vi "Scripting_GetControlFromTypeDef.vi"(0 "TypeDefControl":path=path "C:/classes/ObjectAttributes.ctl", 1 "String":string="Base class.Base class.Attribute1", 5 "error in":errorcluster, 6 "AppRef":refnum<vi>) -> (14 "vi reference":refnum<vi>, 15 "Panel":refnum<vi>, 16 "ControlRef":refnum<vi>, 19 "error out":errorcluster)   [LabVIEW 2020]
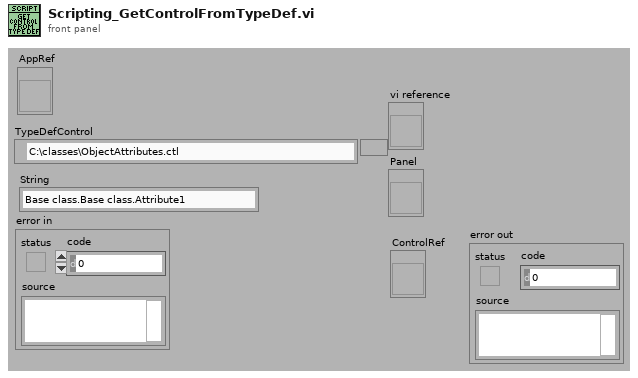
[diagram p1: front panel]
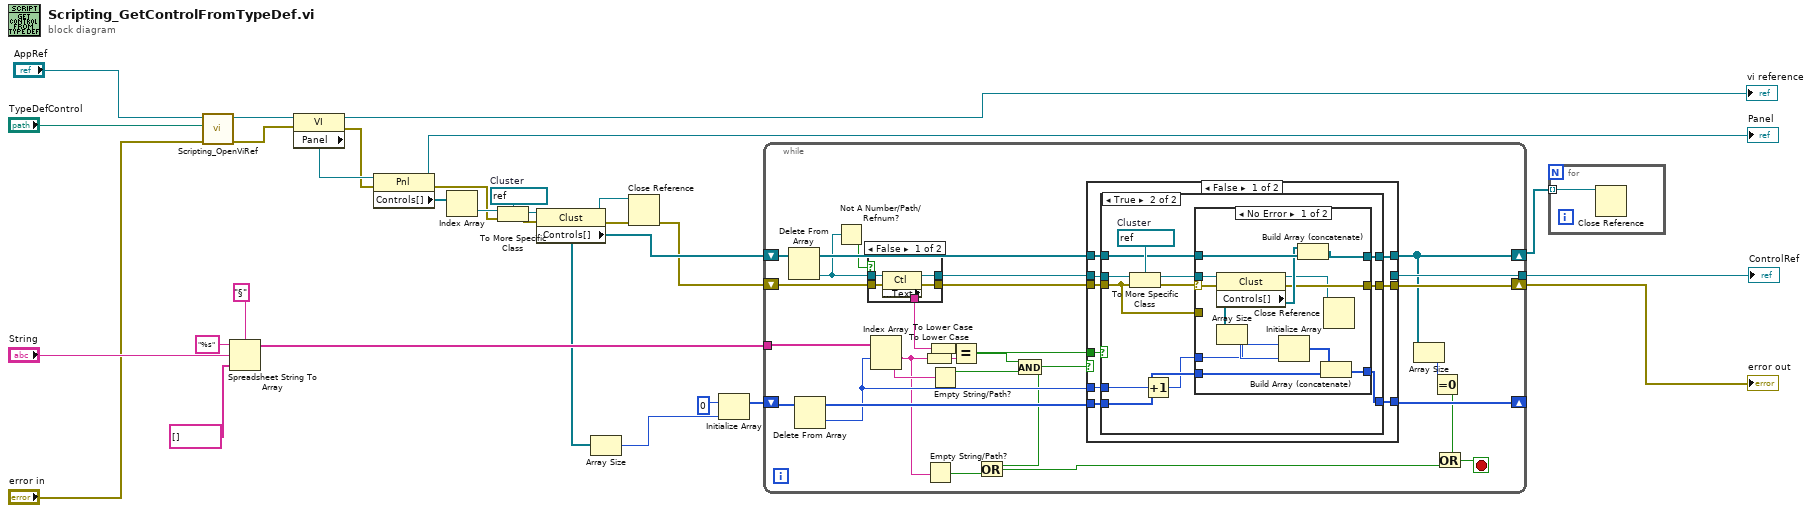
[diagram p0: block diagram]
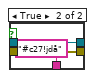
[diagram p2: hidden frame]
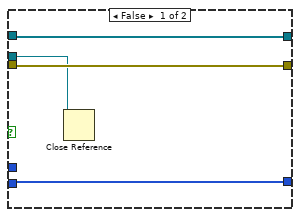
[diagram p3: hidden frame]
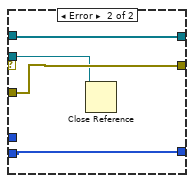
[diagram p4: hidden frame]
diagram:
  w27 = refnum<vi> refnum  # Cluster
  n1 = call <resource>:"Scripting_OpenViRef.vi"("error in"="error in", "ViPath/ViName/Viref"="TypeDefControl", "AppRef"="AppRef") -> ("error out"=w7:errorcluster, "vi reference"=w8:refnum<vi>)  [unwired: 6 in, 1 out]
  n2 = Spreadsheet String To Array(delimiter (Tab)="§", format string="%s", spreadsheet string="String", array type (2D Dbl)=string[] []) -> (array=w21:string[])
  n3 = property class="VI"(reference=w8, error in=w7) -> (reference out=→"vi reference":refnum<vi>, error out=w11:errorcluster, "Panel"=w30:refnum<vi>)
  n4 = property class="Pnl"(reference=w30, error in=w11) -> (reference out=→"Panel":refnum<vi>, error out=w10:errorcluster, "Controls[]"=w29:refnum<vi>[])
  n5 = Index Array(array=w29) -> (element=w28:refnum<vi>)  [unwired: 1 in]
  n6 = To More Specific Class(target class=w27, reference=w28, error in=w10) -> (specific class reference=w26:refnum<vi>, error out=w9:errorcluster)
  n7 = property class="Clust"(reference=w26, error in=w9) -> (reference out=w13:refnum<vi>, error out=w14:errorcluster, "Controls[]"=w17:refnum<vi>[])
  n8 = Array Size(array=w17) -> (size(s)=w16:i32)
  n9 = Close Reference(reference=w13, error in (no error)=w14) -> (error out=w2:errorcluster)
  n10 = Initialize Array(0, w16) -> (w19:i32[])
  n11 = while {
    shift-right: [w38] -> w15
    shift-left: w17 -> [w58]
    tunnel: w21 -> [w57]
    shift-right: [w48] -> _
    shift-left: w19 -> [w51]
    tunnel: [w52] -> w20
    shift-right: [w41] -> w3
    shift-left: w2 -> [w43]
    stop <- w39 stop-if-true
    n12 = Delete From Array(array=w58) -> (deleted portion=w35:refnum<vi>, array with subset deleted=w54:refnum<vi>[])  [unwired: 2 in]
    n13 = Delete From Array(array=w51) -> (deleted portion=w49:i32, array with subset deleted=w50:i32[])  [unwired: 2 in]
    n14 = Not A Number/Path/Refnum?(number/path/refnum=w35) -> (NaN/Path/Refnum?=w34:bool)
    n15 = case shown="False" w34 {
      tunnel: [w63 "#c27!jdå" ("Label.Text")] -> w33
      tunnel: [w62 w66] -> w53
      tunnel: w43 -> [w61 w65]
      tunnel: [w60 w65] -> w42
      tunnel: w35 -> [w59 w66]
      frame False {
        n16 = property class="Ctl"(reference=w59, error in=w61) -> (reference out=w62:refnum<vi>, error out=w60:errorcluster, "Label.Text"=w63:string)
      }
      frame True {
      }
    }
    n17 = Index Array(array=w57, index #1=w49) -> (element #1=w46:string, element #2=w56:string)  [unwired: 1 in]
    n18 = To Lower Case(string=w46) -> (all lower case string=w31:string)
    n19 = Empty String/Path?(string/path=w46) -> (empty?=w45:bool)
    n20 = To Lower Case(string=w33) -> (all lower case string=w32:string)
    n21 = Empty String/Path?(string/path=w56) -> (empty?=w55:bool)
    n22 = Equal?(x=w32, y=w31) -> (x = y?=w44:bool)
    n23 = And(x=w44, y=w55) -> (x .and. y?=w47:bool)
    n24 = Or(x=w47, y=w45) -> (x .or. y?=w40:bool)
    n25 = case shown="False" w47 {
      tunnel: w54 -> [w74 w111]
      tunnel: [w73 w111] -> w38
      tunnel: w53 -> [w75 w110]
      tunnel: [_ w110] -> w52
      tunnel: w50 -> [w72 w109]
      tunnel: w49 -> [w71 _]
      tunnel: [w70 w109] -> w48
      tunnel: w44 -> [w69 _]
      tunnel: w42 -> [w68 w108]
      tunnel: [w67 w108] -> w41
      frame False {
        n26 = case shown="True" w69 {
          tunnel: w75 -> [w76 w90]
          tunnel: w74 -> [w79 w87]
          tunnel: [w79 w86] -> w73
          tunnel: w72 -> [w78 w85]
          tunnel: w71 -> [_ w84]
          tunnel: [w78 w82] -> w70
          tunnel: w68 -> [w77 w80]
          tunnel: [w77 w81] -> w67
          frame False {
            n27 = Close Reference(reference=w76) -> ()  [unwired: 1 in, 1 out]
          }
          frame True {
            w91 = refnum<vi> refnum  # Cluster
            n28 = To More Specific Class(target class=w91, reference=w90, error in=w80) -> (specific class reference=w88:refnum<vi>, error out=w89:errorcluster)
            n29 = Increment(x=w84) -> (x+1=w83:i32)
            n30 = case shown="No Error" w89 {
              selector: w89 -> [w103 _]
              tunnel: w88 -> [w102 w104]
              tunnel: w87 -> [w101 w107]
              tunnel: [w100 w107] -> w86
              tunnel: w85 -> [w96 w106]
              tunnel: w83 -> [w97 _]
              tunnel: [w95 w106] -> w82
              tunnel: [w93 w105] -> w81
              tunnel: w80 -> [_ w105]
              frame No Error {
                n31 = property class="Clust"(reference=w102, error in=w103) -> (reference out=w92:refnum<vi>, error out=w93:errorcluster, "Controls[]"=w99:refnum<vi>[])
                n32 = Array Size(array=w99) -> (size(s)=w98:i32)
                n33 = Initialize Array(w97, w98) -> (w94:i32[])
                n34 = Build Array (concatenate)(w99, w101) -> (w100:refnum<vi>[])
                n35 = Build Array (concatenate)(w94, w96) -> (w95:i32[])
                n36 = Close Reference(reference=w92) -> ()  [unwired: 1 in, 1 out]
              }
              frame Error {
                n37 = Close Reference(reference=w104) -> ()  [unwired: 1 in, 1 out]
              }
            }
          }
        }
      }
      frame True {
      }
    }
    n38 = Array Size(array=w38) -> (size(s)=w37:i32)
    n39 = Equal To 0?(x=w37) -> (x = 0?=w36:bool)
    n40 = Or(x=w36, y=w40) -> (x .or. y?=w39:bool)
  }
  "error out" <- w3
  "ControlRef" <- w20
  n41 = for {
    tunnel: w15 -> [w112] mode=indexing
    n42 = Close Reference(reference=w112) -> ()  [unwired: 1 in, 1 out]
  }
